vi "listen.vi"(6 "timeout ms (10000)":i32=10000, 8 "error in":errorcluster, 11 "connection server in":refnum<class "connection server.lvclass">) -> (0 "error out":errorcluster, 1 "valid?":bool, 2 "new connection":refnum<class "connection maintainer.lvclass">, 3 "connection server out":refnum<class "connection server.lvclass">, 5 "client ID":string)   [LabVIEW 2015, in "connection server.lvclass"]
uses:
  connection server.lvclass
  connection/connection maintainer.lvclass
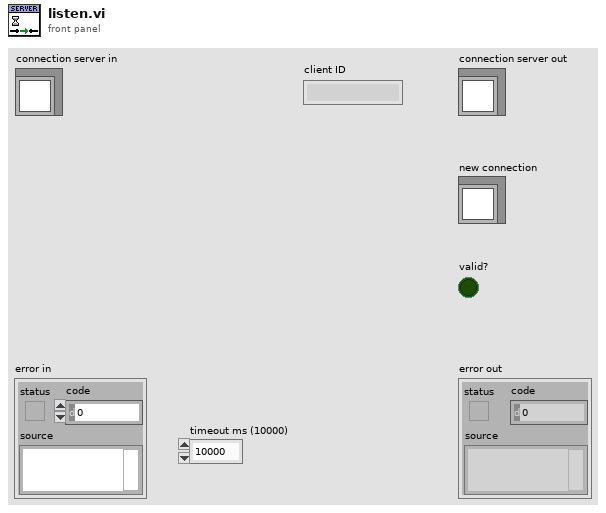
[diagram p1: front panel]
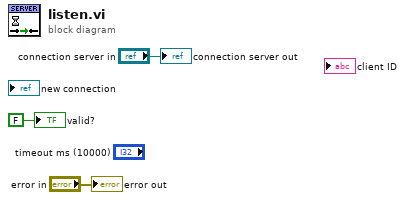
[diagram p0: block diagram]
diagram:
  "error out" <- "error in"
  "connection server out" <- "connection server in"
  "valid?" <- FALSE ("valid?")
